vi "Add Session.vi"(6 "instrument type id":string, 7 "session to add":variant, 8 "error in":errorcluster, 9 "site":i32, 10 "pin or relay name":string, 11 "connection map in":refnum<class "Connection Map.lvclass">) -> (0 "error out":errorcluster, 3 "connection map out":refnum<class "Connection Map.lvclass">)   [LabVIEW 2020, in "Plug-In SDK Session Management V1 API.lvlib" / "Connection Map.lvclass"]
uses:
  Connection Map.lvclass
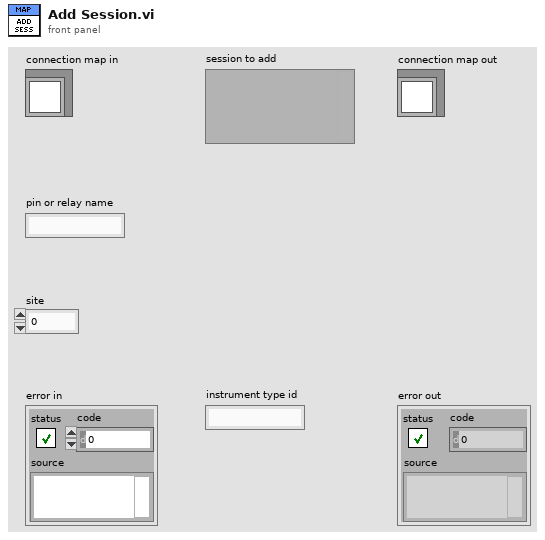
[diagram p1: front panel]
types:
  T1 = typedef "Plug-In SDK Session Management V1 API.lvlib/Session Reservation.lvclass/Connection with Session.ctl" = cluster{"connection":T2, "session":variant}
  T2 = typedef "Plug-In SDK Session Management V1 API.lvlib/Session Reservation.lvclass/Connection.ctl" = cluster{"pin or relay name":string, "site":i32, "instrument type id":string, "channel":string}
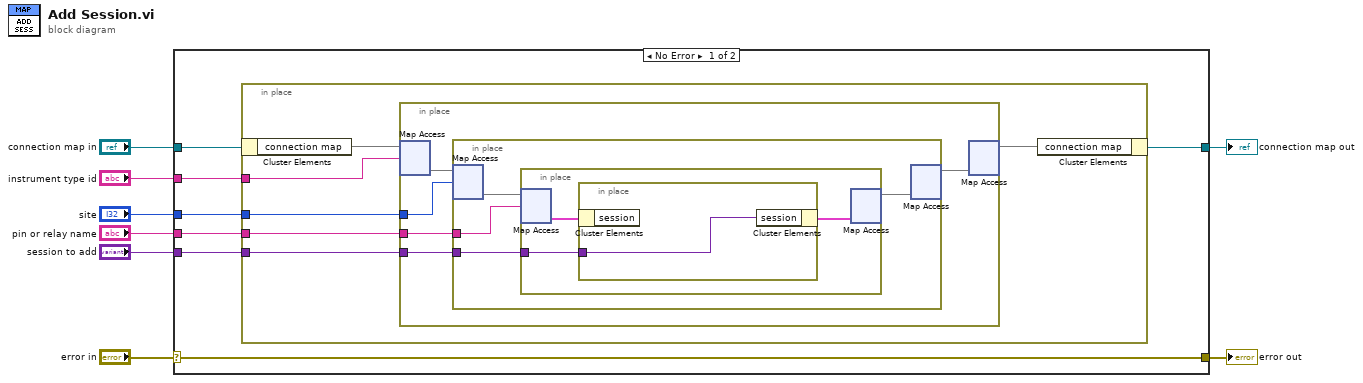
[diagram p0: block diagram]
diagram:
  n1 = case shown="No Error" "error in" {
    selector: "error in" -> [w15 w36]
    tunnel: [w15 w36] -> w7
    tunnel: [w10 w35] -> w5
    tunnel: "connection map in" -> [w14 w35]
    tunnel: "instrument type id" -> [w13 _]
    tunnel: "site" -> [w12 _]
    tunnel: "pin or relay name" -> [w11 _]
    tunnel: "session to add" -> [w9 _]
    frame No Error {
      n2 = in-place {
        in-place-border: w13 -> [w20]
        in-place-border: w12 -> [w19]
        in-place-border: w11 -> [w18]
        in-place-border: w9 -> [w16]
        n3 = in-place-cluster #1(w14) -> ("connection map"=w21:map{string, map{i32, map{string, T1}}})
        n4 = in-place {
          in-place-border: w19 -> [w25]
          in-place-border: w18 -> [w24]
          in-place-border: w16 -> [w22]
          n5 = in-place-map #2(w21, w20) -> (w26:map{i32, map{string, T1}})  [unwired: 1 in, 1 out]
          n6 = in-place {
            in-place-border: w24 -> [w29]
            in-place-border: w22 -> [w27]
            n7 = in-place-map #3(w26, w25) -> (w30:map{string, T1})  [unwired: 1 in, 1 out]
            n8 = in-place {
              in-place-border: w27 -> [w31]
              n9 = in-place-map #4(w30, w29) -> (w33:T1)  [unwired: 1 in, 1 out]
              n10 = in-place {
                in-place-border: w31 -> [w34]
                n11 = in-place-cluster #5(w33) -> ()  [unwired: 1 out]
                n12 = in-place-cluster #5("session"=w34) -> (w32:T1)
              }
              n13 = in-place-map #4(w32) -> (w28:map{string, T1})  [unwired: 1 in, 2 out]
            }
            n14 = in-place-map #3(w28) -> (w23:map{i32, map{string, T1}})  [unwired: 1 in, 2 out]
          }
          n15 = in-place-map #2(w23) -> (w17:map{string, map{i32, map{string, T1}}})  [unwired: 1 in, 2 out]
        }
        n16 = in-place-cluster #1("connection map"=w17) -> (w10:refnum<class "Connection Map.lvclass">)
      }
    }
    frame Error {
    }
  }
  "error out" <- w7
  "connection map out" <- w5
